vi "MHL_get analysis parameters.vi"(0 "Data Cluster in":T2, 1 "Get analysis parameters Argument":T1, 5 "error in (no error)":errorcluster) -> (14 "Data Cluster out":T2, 19 "error out":errorcluster)   [LabVIEW 2019, in "Main UI.lvlib"]
uses:
  Main UI.lvlib
  Module Data--cluster.ctl
  Class Library/XYgraph_class/XYgraph.lvclass
  FileReader/FPref_clustered--cluster references.ctl
  Main UI Shared/Boolean--FP cluster.ctl
  FileReader/FPref_cntrls--cluster references.ctl
  Main UI Shared/Indicators--FP cluster.ctl
  Get analysis parameters Argument--cluster.ctl
  Get analysis parameters (Reply Payload)--cluster.ctl
  Main UI Shared/Decimation input --cluster.ctl
  Main UI Shared/MAIN UI Shared.lvlib
panel:
  # "Contact"
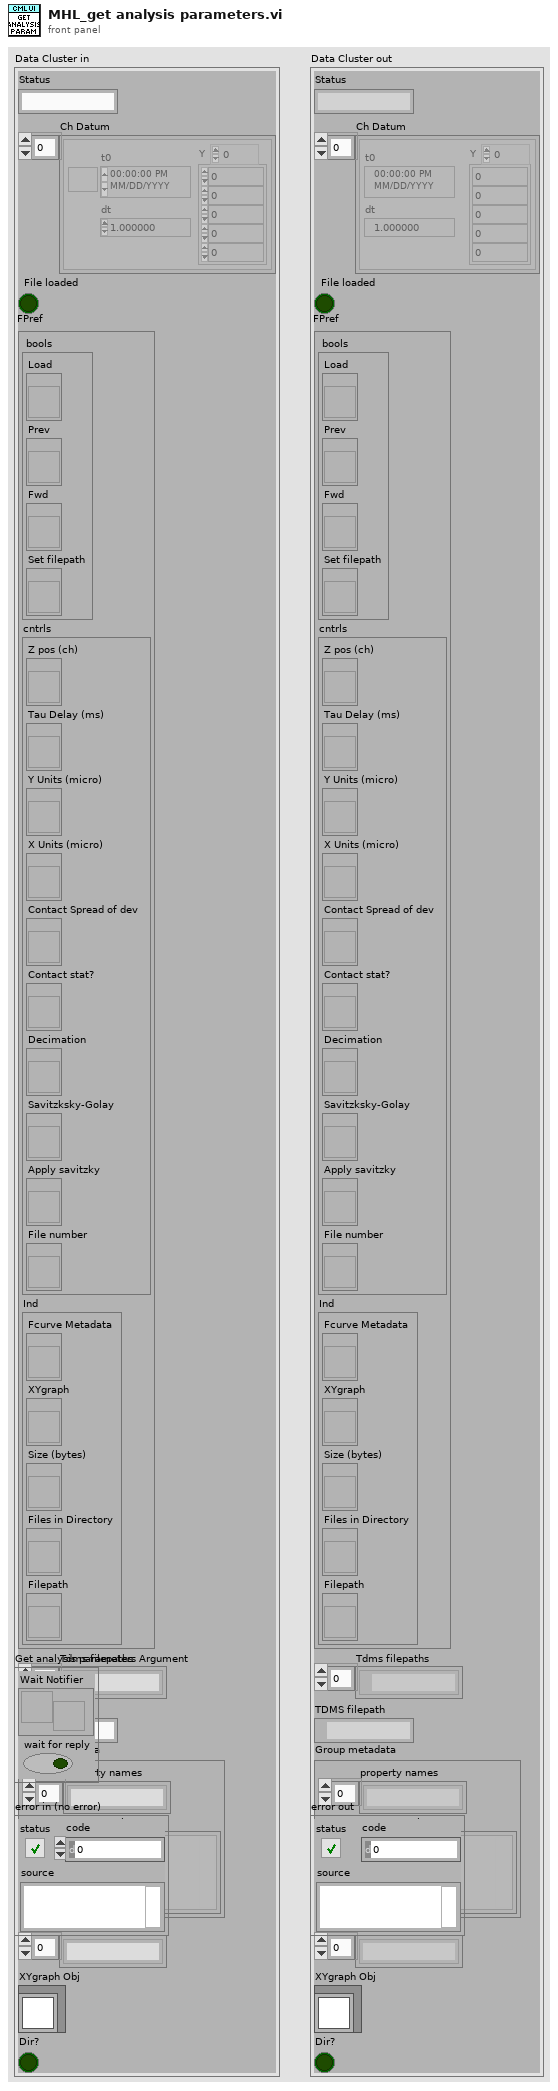
[diagram p1: front panel]
types:
  T1 = typedef "Main UI.lvlib/Get analysis parameters Argument--cluster.ctl" = cluster{"Wait Notifier":refnum<notifier>, "wait for reply":bool}
  T2 = typedef "Main UI.lvlib/Module Data--cluster.ctl" = cluster{"Status":string, "Ch Datum":waveform(dbl)[], "File loaded":bool, "FPref":T3, "Tdms filepaths":path[], "TDMS filepath":path, "Group metadata":cluster{"property names":string[], "property values":variant[]}, "Channel name(s)":string[], "XYgraph Obj":refnum<class "XYgraph.lvclass">, "Dir?":bool}
  T3 = typedef "Main UI.lvlib/FPref_clustered--cluster references.ctl" = cluster{" bools":T4, "cntrls":T5, "Ind":T6}
  T4 = typedef "MAIN UI Shared.lvlib/Boolean--FP cluster.ctl" = cluster{"Load":refnum<vi>, "Prev":refnum<vi>, "Fwd":refnum<vi>, "Set filepath":refnum<vi>}
  T5 = typedef "Main UI.lvlib/FPref_cntrls--cluster references.ctl" = cluster{"Z pos (ch)":refnum<vi>, "Tau Delay (ms)":refnum<vi>, "Y Units (micro)":refnum<vi>, "X Units (micro)":refnum<vi>, "Contact Spread of dev":refnum<vi>, "Contact stat?":refnum<vi>, "Decimation":refnum<vi>, "Savitzksky-Golay":refnum<vi>, "Apply savitzky ":refnum<vi>, "File number":refnum<vi>}
  T6 = typedef "Main UI.lvlib/Indicators--FP cluster.ctl" = cluster{"Fcurve Metadata":refnum<vi>, "XYgraph":refnum<vi>, "Size (bytes)":refnum<vi>, "Files in Directory":refnum<vi>, "Filepath":refnum<vi>}
  T7 = cluster{"Contact stat?":bool, "Contact Spread of dev":dbl}
  T8 = typedef "Main UI.lvlib/Get analysis parameters (Reply Payload)--cluster.ctl" = cluster{"Contact":cluster{"Contact stat?":bool, "Contact Spread of dev":dbl}, "Decimation":T9, "Savitzksky-Golay":cluster{"Sidepoints (M)":dbl, "Filter Order":i32}, "Tau Delay (ms)":dbl, "error":errorcluster}
  T9 = typedef "MAIN UI Shared.lvlib/Decimation input --cluster.ctl" = cluster{"App":cluster{"Dec":i32, "apply":bool}, "Con":cluster{"Dec":i32, "apply":bool}, "Ret":cluster{"Dec":i32, "apply":bool}}
  T10 = cluster{"Sidepoints (M)":dbl, "Filter Order":i32}
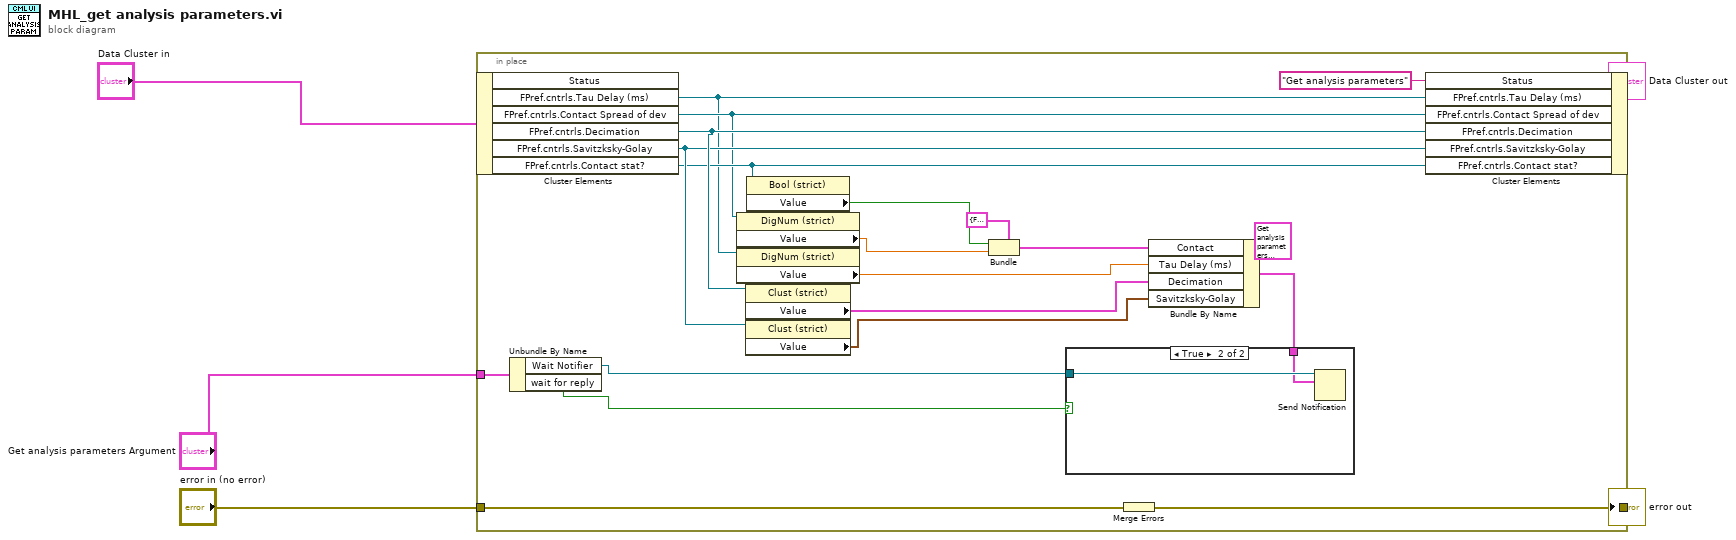
[diagram p0: block diagram]
diagram:
  n1 = in-place {
    in-place-border: "error in (no error)" -> [w25]
    in-place-border: "Get analysis parameters Argument" -> [w24]
    in-place-border: [w19] -> w3
    n2 = in-place-cluster #1("Data Cluster in") -> ("FPref.cntrls.Tau Delay (ms)"=w9:refnum<vi>, "FPref.cntrls.Contact Spread of dev"=w10:refnum<vi>, "FPref.cntrls.Decimation"=w17:refnum<vi>, "FPref.cntrls.Savitzksky-Golay"=w16:refnum<vi>, "FPref.cntrls.Contact stat?"=w14:refnum<vi>)  [unwired: 1 out]
    n3 = Unbundle By Name(w24) -> ("Wait Notifier"=w23:refnum<notifier>, "wait for reply"=w22:bool)
    n4 = property class="DigNum (strict)"(reference=w10) -> ("Value"=w12:dbl)  [unwired: 1 in, 2 out]
    n5 = property class="DigNum (strict)"(reference=w9) -> ("Value"=w8:dbl)  [unwired: 1 in, 2 out]
    n6 = property class="Clust (strict)"(reference=w17) -> ("Value"=w7:T9)  [unwired: 1 in, 2 out]
    n7 = property class="Clust (strict)"(reference=w16) -> ("Value"=w6:T10)  [unwired: 1 in, 2 out]
    n8 = property class="Bool (strict)"(reference=w14) -> ("Value"=w13:bool)  [unwired: 1 in, 2 out]
    n9 = Bundle(cluster=T7 {"Contact stat?"=FALSE, "Contact Spread of dev"=0.0} ("Contact"), "Contact stat?"=w13, "Contact Spread of dev"=w12) -> (w11:T7)
    n10 = Merge Errors(w25) -> (w19:errorcluster)
    n11 = Bundle By Name(cluster=T8 {"Contact"={"Contact stat?"=TRUE, "Contact Spread of dev"=0.0}, "Decimation"={"App"={"Dec"=1, "apply"=FALSE}, "Con"={"Dec"=1, "apply"=FALSE}, "Ret"={"Dec"=1, "apply"=FALSE}}, "Savitzksky-Golay"={"Sidepoints (M)"=20.0, "Filter Order"=5}, "Tau Delay (ms)"=0.0, "error"={"status"=FALSE, "code"=0, "source"=""}} ("Get analysis parameters (Reply Payload)"), "Contact"=w11, "Tau Delay (ms)"=w8, "Decimation"=w7, "Savitzksky-Golay"=w6) -> (w21:T8)
    n12 = case shown="True" w22 {
      tunnel: w23 -> [_ w27]
      tunnel: w21 -> [_ w26]
      frame False {
      }
      frame True {
        n13 = Send Notification(notification=w26, notifier=w27) -> ()  [unwired: 1 in, 2 out]
      }
    }
    n14 = in-place-cluster #1("Status"="Get analysis parameters", "FPref.cntrls.Tau Delay (ms)"=w9, "FPref.cntrls.Contact Spread of dev"=w10, "FPref.cntrls.Decimation"=w17, "FPref.cntrls.Savitzksky-Golay"=w16, "FPref.cntrls.Contact stat?"=w14) -> (→"Data Cluster out":T2)
  }
  "error out" <- w3
